vi "_Default Instrument Setup.vi"(8 "error in (no error)":errorcluster, 11 "VISA resource name":refnum<visa-resource-name>) -> (0 "error out":errorcluster, 3 "VISA resource name out":refnum<visa-resource-name>)   [LabVIEW 2015, in "Rohde&Schwarz CMXP Base.lvlib"]
doc: "This Utility VI sends a default command string to the instrument whenever a new VISA session is opened, or the instrument is reset.\nThis VI is intended to be used as a subVI for the Initialize.vi and Reset VI. Altering this VI could cause these two VI's to operate incorrectly."
uses:
  <instrlib>/Rohde&Schwarz CMXP Base/Rohde&Schwarz CMXP Base.lvlib
  <instrlib>/Rohde&Schwarz CMXP Base/Private/rsidr_core.llb/type_Options_Item_Parsing.ctl
  <instrlib>/Rohde&Schwarz CMXP Base/Private/rsidr_core.llb/rsidr_core.lvlib
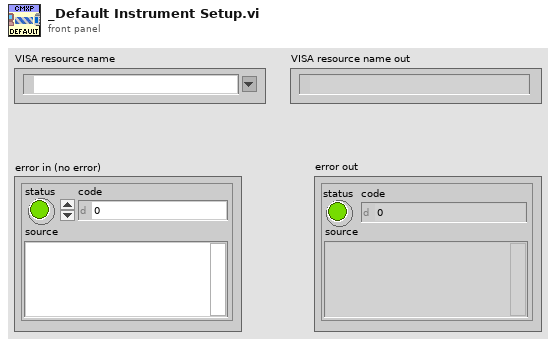
[diagram p1: front panel]
types:
  T1 = typedef "Rohde&Schwarz CMXP Base.lvlib/rsidr_core.lvlib/type_Options_Item_Parsing.ctl" = enum16{"None", "Keep parts after dash", "Keep parts before dash", "Automatic"}
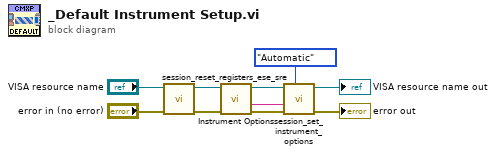
[diagram p0: block diagram]
diagram:
  n1 = call <instrlib>:"session_reset_registers_ese_sre.vi"("error in"="error in (no error)", "VISA resource name"="VISA resource name") -> ("error out"=w4:errorcluster, "VISA resource name out"=w3:refnum<visa-resource-name>)  [unwired: 8 in]
  n2 = call <instrlib>:"Instrument Options.vi"("error in (no error)"=w4, "VISA resource name"=w3) -> ("error out"=w10:errorcluster, "Options List"=w7:string, "VISA resource name out"=w2:refnum<visa-resource-name>)  [unwired: 7 in]
  n3 = call <instrlib>:"session_set_instrument_options.vi"("Item Parsing"=type_Options_Item_Parsing."Automatic", "error in"=w10, "Options string"=w7, "VISA resource name"=w2) -> ("error out"=→"error out":errorcluster, "VISA resource name out"=→"VISA resource name out":refnum<visa-resource-name>)  [unwired: 4 in, 2 out]
